vi "Image for Use_0 (1).vi"(7 "Command":enum16{"Create", "Use", "Copy in", "Dispose"}(ring)=enum."Use", 8 "error in":errorcluster, 10 "Image Type":T1=4 items=["Grayscale (U8)", "Grayscale (I16)", "Grayscale (SGL)", "Complex (CSG)", "RGB (U32)", "HSL (U32)", "RGB (U64)", "Grayscale (U16)"], 11 "Image Src":T2) -> (0 "error out":errorcluster, 3 "Image out":T2)   [LabVIEW 2015]
uses:
  <vilib>/vision/Image Controls.llb/IMAQ Image.ctl
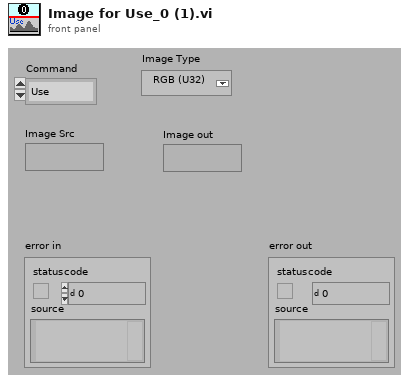
[diagram p1: front panel]
types:
  T1 = typedef "Image Type" = u32
  T2 = typedef "IMAQ Image.ctl" = refnum<image>
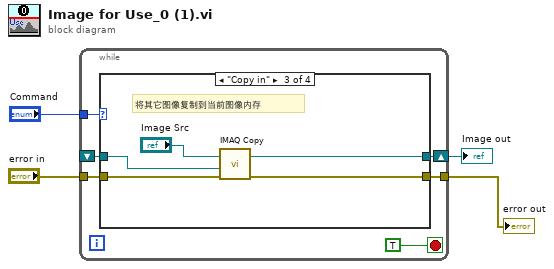
[diagram p0: block diagram]
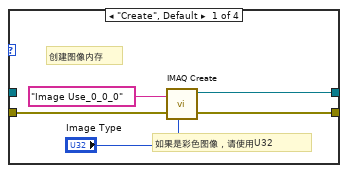
[diagram p2: hidden frame]
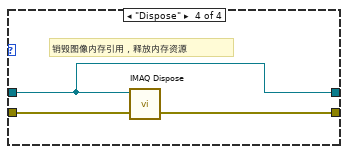
[diagram p4: hidden frame]
diagram:
  n1 = while {
    tunnel: "Command" -> [w10]
    tunnel: "error in" -> [w9]
    tunnel: [w8] -> w1
    shift-right: [w7] -> w2
    shift-left: _ -> [w6]
    stop <- TRUE stop-if-true
    n2 = case shown="\"Copy in\"" w10 {
      tunnel: w9 -> [w14 w17 w21 w25]
      tunnel: [w13 w17 w20 w24] -> w8
      tunnel: [w12 w16 w22 w23] -> w7
      tunnel: w6 -> [_ w16 w18 w23]
      frame "Create", Default {
        # "如果是彩色图像，请使用U32"
        # "创建图像内存"
        n3 = call "IMAQ Create"("Image Name"="Image Use_0_0_0", "Image Type"="Image Type", "error in (no error)"=w14) -> ("New Image"=w12:T2, "error out"=w13:errorcluster)  [unwired: 1 in, 1 out]
      }
      frame "Use" {
        # "使用图像内存"
      }
      frame "Copy in" {
        # "将其它图像复制到当前图像内存"
        n4 = call "IMAQ Copy"("error in (no error)"=w21, "Image Dst"=w18, "Image Src"="Image Src") -> ("error out"=w20:errorcluster, "Image Dst Out"=w22:T2)  [unwired: 3 out]
      }
      frame "Dispose" {
        # "销毁图像内存引用，释放内存资源"
        n5 = call "IMAQ Dispose"("Image"=w23, "error in (no error)"=w25) -> ("error out"=w24:errorcluster)  [unwired: 1 in, 3 out]
      }
    }
  }
  "Image out" <- w2
  "error out" <- w1
